vi "Launching.vi"(8 "error in (no error)":errorcluster, 11 "BuildServer in":refnum<class "BuildServer.lvclass">) -> (0 "error out":errorcluster, 3 "BuildServer out":refnum<class "BuildServer.lvclass">)   [LabVIEW 2017, in "BuildServer.lvlib" / "BuildServer.lvclass"]
uses:
  BuildServer.lvclass
  <vilib>/ActorFramework/Actor/Actor.lvclass
  BuildServer Messages/Reset UI Msg/Reset UI Msg.lvclass
  BuildServer Messages/Launch Nested Actors Msg/Launch Nested Actors Msg.lvclass
  BuildServer Messages/Launch New Worker Msg/Launch New Worker Msg.lvclass
  WebSocket Server/Actors/Actor wHelper/Actor wLauncher Messages/Send Message to Launcher Msg/Send Message to Launcher Msg.lvclass
  WebSocket Server/Actors/Actor wHelper/Actor wLauncher Messages/Close Launcher Msg/Close Launcher Msg.lvclass
  WebSocket Server/Actors/Actor wHelper/Actor wUI Messages/Show UI Msg/Show UI Msg.lvclass
  Volumes/Data/Users/benji667/Git/BuildFarm/WebSocket Server/Actors/Actor wHelper/Actor wHelper/Actor wHelper.lvclass
  Volumes/Data/Users/benji667/Git/BuildFarm/WebSocket Server/Actors/Actor wHelper/Actor wLauncher/Actor wLauncher.lvclass
  Volumes/Data/Users/benji667/Git/BuildFarm/WebSocket Server/Actors/Actor wHelper/Actor wUI/Actor wUI.lvclass
  Applications/National Instruments/LabVIEW 2017 64-bit/vi.lib/ActorFramework/Actor/Actor.lvclass
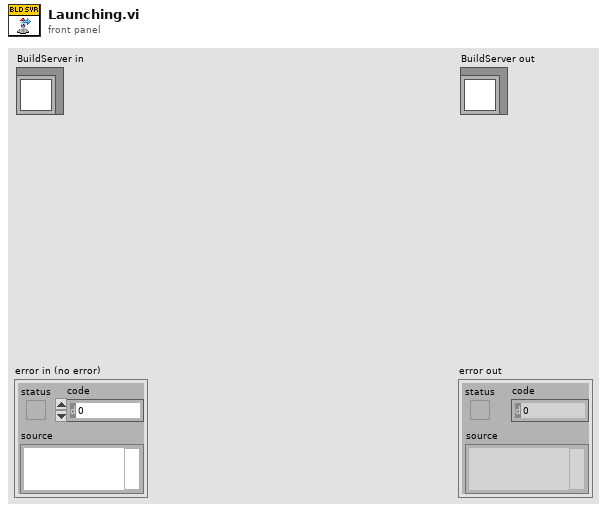
[diagram p1: front panel]
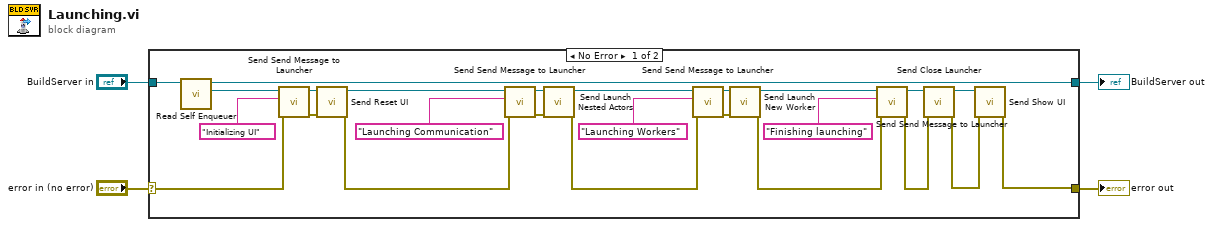
[diagram p0: block diagram]
diagram:
  n1 = case shown="No Error" "error in (no error)" {
    selector: "error in (no error)" -> [w19 w30]
    tunnel: [w5 w30] -> w3
    tunnel: [w28 w29] -> w1
    tunnel: "BuildServer in" -> [w28 w29]
    frame No Error {
      n2 = call <vilib>:"Read Self Enqueuer.vi"("Actor"=w28) -> ("Self Enqueuer"=w27:refnum<class "Message Enqueuer.lvclass">)  [unwired: 10 in]
      n3 = call "Send Send Message to Launcher.vi"("error in (no error)"=w19, "Msg to Launcher"="Initializing UI", "Message Enqueuer"=w27) -> ("error out"=w18:errorcluster, "Message Enqueuer out"=w26:refnum<class "Message Enqueuer.lvclass">)  [unwired: 7 in]
      n4 = call "Send Reset UI.vi"("error in (no error)"=w18, "Message Enqueuer"=w26) -> ("error out"=w17:errorcluster, "Message Enqueuer out"=w25:refnum<class "Message Enqueuer.lvclass">)  [unwired: 8 in]
      n5 = call "Send Send Message to Launcher.vi"("error in (no error)"=w17, "Msg to Launcher"="Launching Communication", "Message Enqueuer"=w25) -> ("error out"=w16:errorcluster, "Message Enqueuer out"=w24:refnum<class "Message Enqueuer.lvclass">)  [unwired: 7 in]
      n6 = call "Send Launch Nested Actors.vi"("error in (no error)"=w16, "Message Enqueuer"=w24) -> ("error out"=w15:errorcluster, "Message Enqueuer out"=w23:refnum<class "Message Enqueuer.lvclass">)  [unwired: 8 in]
      n7 = call "Send Send Message to Launcher.vi"("error in (no error)"=w15, "Msg to Launcher"="Launching Workers", "Message Enqueuer"=w23) -> ("error out"=w14:errorcluster, "Message Enqueuer out"=w22:refnum<class "Message Enqueuer.lvclass">)  [unwired: 7 in]
      n8 = call "Send Launch New Worker.vi"("error in (no error)"=w14, "Message Enqueuer"=w22) -> ("error out"=w13:errorcluster, "Message Enqueuer out"=w21:refnum<class "Message Enqueuer.lvclass">)  [unwired: 8 in]
      n9 = call "Send Send Message to Launcher.vi"("error in (no error)"=w13, "Msg to Launcher"="Finishing launching", "Message Enqueuer"=w21) -> ("error out"=w12:errorcluster, "Message Enqueuer out"=w20:refnum<class "Message Enqueuer.lvclass">)  [unwired: 7 in]
      n10 = call "Send Close Launcher.vi"("error in (no error)"=w12, "Message Enqueuer"=w20) -> ("error out"=w6:errorcluster, "Message Enqueuer out"=w7:refnum<class "Message Enqueuer.lvclass">)  [unwired: 8 in]
      n11 = call "Send Show UI.vi"("error in (no error)"=w6, "Message Enqueuer"=w7) -> ("error out"=w5:errorcluster)  [unwired: 8 in, 1 out]
    }
    frame Error {
    }
  }
  "error out" <- w3
  "BuildServer out" <- w1
